vi "set_current.vi"(8 "error in":errorcluster, 10 "current":dbl, 11 "VISA resource name":refnum<visa-resource-name>="COM1") -> (0 "error out":errorcluster, 3 "VISA resource name out":refnum<visa-resource-name>)   [LabVIEW 2020]
panel:
  out "command":string
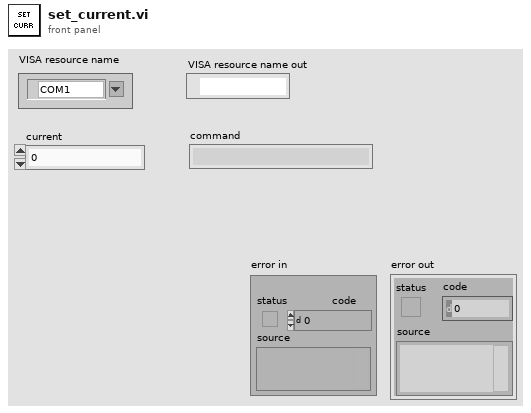
[diagram p1: front panel]
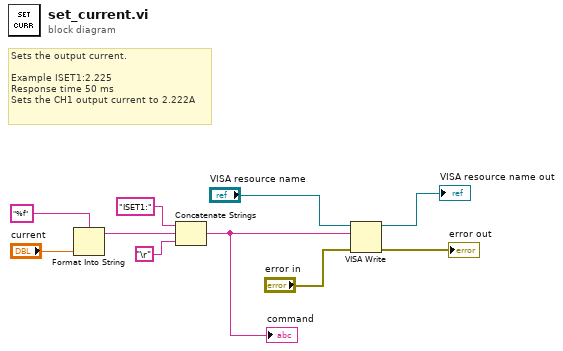
[diagram p0: block diagram]
diagram:
  # "Sets the output current.\n\nExample ISET1:2.225\nResponse time 50 ms\nSets the CH1 output current to 2.222A"
  n1 = Format Into String(format string="%f", "current") -> (resulting string=w9:string)  [unwired: 2 in, 1 out]
  n2 = Concatenate Strings("ISET1:" ("string"), w9, "\r") -> (w4:string)
  "command" <- w4
  n3 = VISA Write(VISA resource name="VISA resource name", write buffer=w4, error in (no error)="error in") -> (VISA resource name out=→"VISA resource name out":refnum<visa-resource-name>, error out=→"error out":errorcluster)  [unwired: 1 out]
